vi "channel.data_source_rid.vi"(8 "error in":errorcluster, 11 "Channel in":refnum<class "Channel.lvclass">) -> (0 "error out":errorcluster, 2 "source rid":string, 3 "Channel out":refnum<class "Channel.lvclass">)   [LabVIEW 2020, in "Channel.lvclass"]
doc: "Returns the RID of the dataset, video, or connection that owns this channel."
uses:
  Channel.lvclass
  Channel.lvclass/Channel.ctl
  client.lvlib
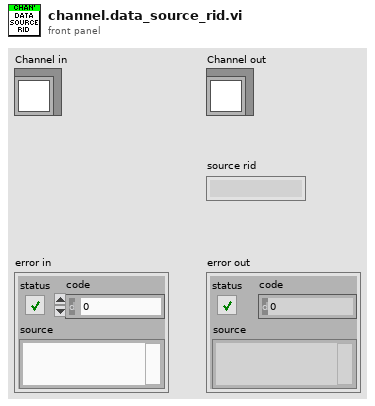
[diagram p1: front panel]
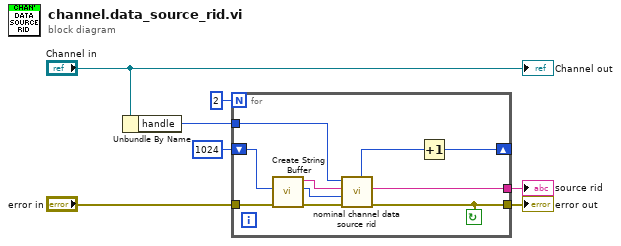
[diagram p0: block diagram]
diagram:
  n1 = Unbundle By Name("Channel in") -> ("handle"=w4:i32)
  n2 = for {
    N: 2 -> [_]
    tunnel: w4 -> [w17]
    tunnel: [w16] -> w1
    shift-right: [w9] -> _
    shift-left: 1024 ("Buffer Size (1024)") -> [w13]
    tunnel: [w10] -> w2
    tunnel: "error in" -> [w8]
    stop <- w10 continue-if-true
    n3 = call "Create String Buffer.vi"("error in"=w8, "Buffer Size (1024)"=w13) -> ("error out"=w12:errorcluster, "dub Buffer Size"=w14:i32, "String Buffer"=w15:string)  [unwired: 7 in]
    n4 = call "nominal channel data source rid.vi"("error in (no error)"=w12, "cap"=w14, "buf"=w15, "channel"=w17) -> ("error out"=w10:errorcluster, "buf out"=w16:string, "out_needed out"=w11:u32)  [unwired: 4 in, 1 out]
    n5 = Increment(x=w11) -> (x+1=w9:u32)
  }
  "error out" <- w2
  "source rid" <- w1
  "Channel out" <- "Channel in"
